vi "Clear-Load Spurious Threshold Data.vi"(7 "Threshold Data File Name ( )":path, 8 "error in (no error)":errorcluster, 9 "Operation (0: Clear Data)":enum16{"Clear Data", "Load Data"}(ring), 10 "Measurement Type (6: Phase Noise)":u16(ring)=6 items=["AM Noise"=1, "Baseband Noise"=2, "Freq/Power"=3, "Spectrum"=4, "Transient"=5, "Phase Noise"=6, "User"=7], 11 "VISA resource name":refnum<visa-resource-name>) -> (0 "error out":errorcluster, 3 "VISA resource name out":refnum<visa-resource-name>)   [LabVIEW 2011, in "Agilent E5052X.lvlib"]
doc: "Clears or loads user defined threshold data for spurious measurements. \n\n<b>Note: </b>\n\nThis VI only applies to Phase, AM and Baseband noise measurements."
uses:
  Agilent E5052X.lvlib
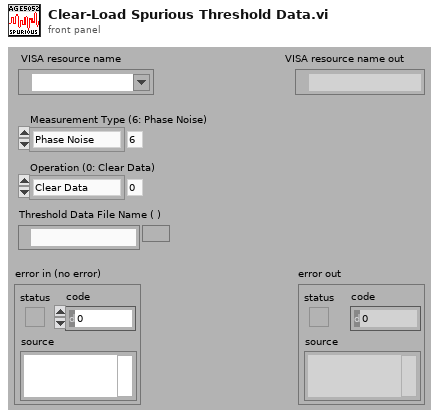
[diagram p1: front panel]
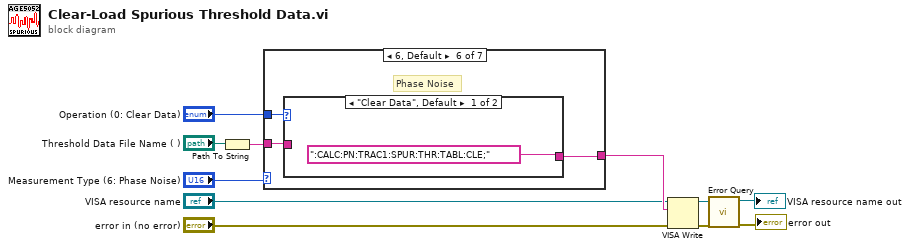
[diagram p0: block diagram]
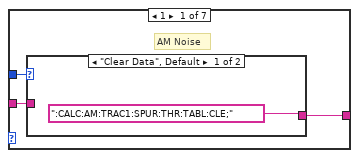
[diagram p2: hidden frame]
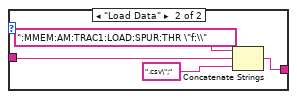
[diagram p3: hidden frame]
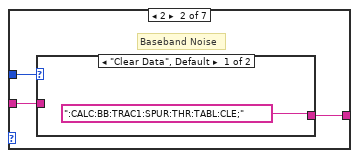
[diagram p4: hidden frame]
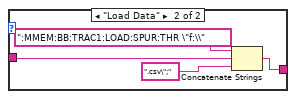
[diagram p5: hidden frame]
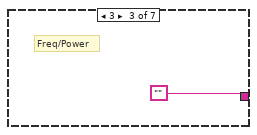
[diagram p6: hidden frame]
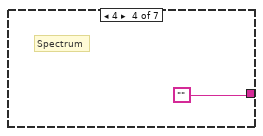
[diagram p7: hidden frame]
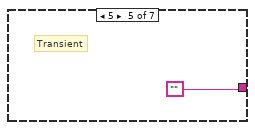
[diagram p8: hidden frame]
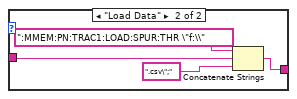
[diagram p9: hidden frame]
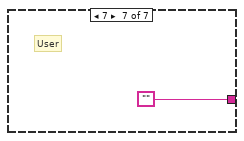
[diagram p10: hidden frame]
diagram:
  n1 = Path To String(path="Threshold Data File Name ( )") -> (string=w1:string)
  n2 = case shown="6, Default" "Measurement Type (6: Phase Noise)" {
    tunnel: "Operation (0: Clear Data)" -> [w14 w22 _ _ _ w33 _]
    tunnel: [w13 w20 "" "" "" w31 ""] -> w10
    tunnel: w1 -> [w12 w21 _ _ _ w32 _]
    frame 1 {
      # "AM Noise"
      n3 = case shown="\"Clear Data\", Default" w14 {
        tunnel: [":CALC:AM:TRAC1:SPUR:THR:TABL:CLE;" w16] -> w13
        tunnel: w12 -> [_ w17]
        frame "Clear Data", Default {
        }
        frame "Load Data" {
          n4 = Concatenate Strings(":MMEM:AM:TRAC1:LOAD:SPUR:THR \"f:\\", w17, ".csv\";" ("string")) -> (w16:string)
        }
      }
    }
    frame 2 {
      # "Baseband Noise"
      n5 = case shown="\"Clear Data\", Default" w22 {
        tunnel: [":CALC:BB:TRAC1:SPUR:THR:TABL:CLE;" w24] -> w20
        tunnel: w21 -> [_ w25]
        frame "Clear Data", Default {
        }
        frame "Load Data" {
          n6 = Concatenate Strings(":MMEM:BB:TRAC1:LOAD:SPUR:THR \"f:\\", w25, ".csv\";" ("string")) -> (w24:string)
        }
      }
    }
    frame 3 {
      # "Freq/Power"
    }
    frame 4 {
      # "Spectrum"
    }
    frame 5 {
      # "Transient"
    }
    frame 6, Default {
      # "Phase Noise"
      n7 = case shown="\"Clear Data\", Default" w33 {
        tunnel: [":CALC:PN:TRAC1:SPUR:THR:TABL:CLE;" w35] -> w31
        tunnel: w32 -> [_ w36]
        frame "Clear Data", Default {
        }
        frame "Load Data" {
          n8 = Concatenate Strings(":MMEM:PN:TRAC1:LOAD:SPUR:THR \"f:\\", w36, ".csv\";" ("string")) -> (w35:string)
        }
      }
    }
    frame 7 {
      # "User"
    }
  }
  n9 = VISA Write(VISA resource name="VISA resource name", write buffer=w10, error in (no error)="error in (no error)") -> (VISA resource name out=w9:refnum<visa-resource-name>, error out=w8:errorcluster)  [unwired: 1 out]
  n10 = call "Error Query.vi"("error in (no error)"=w8, "VISA resource name"=w9) -> ("error out"=→"error out":errorcluster, "VISA resource name out"=→"VISA resource name out":refnum<visa-resource-name>)  [unwired: 6 in, 2 out]
